vi "VariacContoroller(PID).vi"() -> ()   [LabVIEW 2019]
panel:
  out "lower limit":dbl
  out "upper limit":dbl
  out "In Range?":bool
  out "coerced(x)":dbl
  out "Tolearance value":dbl
  in  "Tolearance in percentage":dbl
  out "voltage lower":bool
  out "voltage higher":bool
  in  "Voltage Feedback":dbl
  in  "Voltage Set Point":dbl
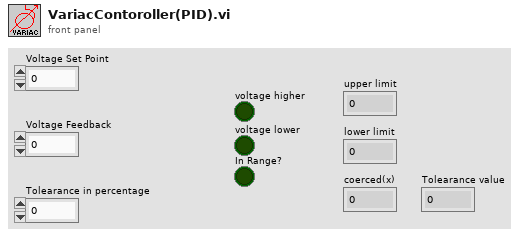
[diagram p1: front panel]
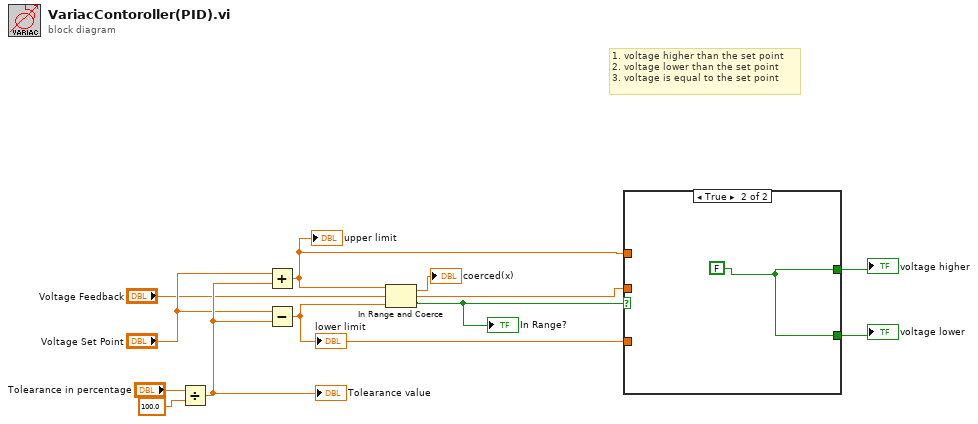
[diagram p0: block diagram]
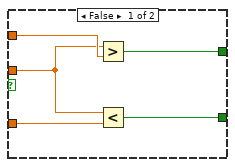
[diagram p2: hidden frame]
diagram:
  # "1. voltage higher than the set point \n2. voltage lower than the set point\n3. voltage is equal to the set point"
  n1 = Divide(x="Tolearance in percentage", y=100.0) -> (x/y=w9:dbl)
  "Tolearance value" <- w9
  n2 = Add(x="Voltage Set Point", y=w9) -> (x+y=w6:dbl)
  "upper limit" <- w6
  n3 = Subtract(x="Voltage Set Point", y=w9) -> (x-y=w5:dbl)
  "lower limit" <- w5
  n4 = In Range and Coerce(upper limit=w6, x="Voltage Feedback", lower limit=w5) -> (coerced(x)=→"coerced(x)":dbl, In Range?=w1:bool)
  "In Range?" <- w1
  n5 = case shown="True" w1 {
    tunnel: w6 -> [w16 _]
    tunnel: w5 -> [w15 _]
    tunnel: "Voltage Feedback" -> [w14 _]
    tunnel: [w13 w17] -> w3
    tunnel: [w12 w17] -> w2
    frame False {
      n6 = Greater?(x=w14, y=w16) -> (0:w12:bool)
      n7 = Less?(x=w14, y=w15) -> (x < y?=w13:bool)
    }
    frame True {
      w17 = FALSE
    }
  }
  "voltage higher" <- w2
  "voltage lower" <- w3
